vi "RSZVB Channel List.vi"(8 "error in (no error)":errorcluster {"code" format="%.0x"}, 11 "VISA session":refnum<visa-resource-name>) -> (0 "error out":errorcluster {"code" format="%.0x"}, 2 "Catalog":string, 3 "dup VISA session":refnum<visa-resource-name>)   [LabVIEW 2011]
doc: "This VI returns the numbers and names of all channels in the current setup.\n\nRemote-control command(s):\nCONFigure:CHANnel<Ch>:CATalog?"
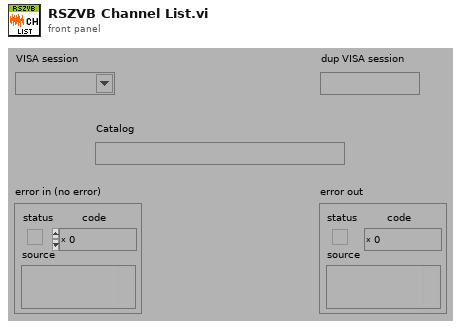
[diagram p1: front panel]
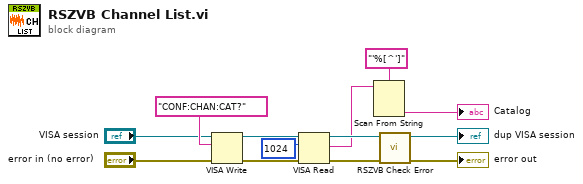
[diagram p0: block diagram]
diagram:
  n1 = VISA Write(VISA resource name="VISA session", write buffer="CONF:CHAN:CAT?", error in (no error)="error in (no error)") -> (VISA resource name out=w12:refnum<visa-resource-name>, error out=w11:errorcluster)  [unwired: 1 out]
  n2 = VISA Read(VISA resource name=w12, byte count=u32 1024 ("byte count (0)"), error in (no error)=w11) -> (VISA resource name out=w5:refnum<visa-resource-name>, read buffer=w2:string, error out=w4:errorcluster)  [unwired: 1 out]
  n3 = Scan From String(format string="'%[^']", input string=w2) -> (output 1=→"Catalog":string)  [unwired: 3 in, 3 out]
  n4 = call "RSZVB Check Error.vi"("error in (no error)"=w4, "VISA session"=w5) -> ("error out"=→"error out":errorcluster, "dup VISA session"=→"dup VISA session":refnum<visa-resource-name>)  [unwired: 8 in]
